vi "LSX Set Stop Accel.vi"(6 "dAD":dbl, 7 "dZD":dbl, 8 "error in (no error)":errorcluster, 9 "dYD":dbl, 10 "dXD":dbl, 11 "lLSID":i32) -> (0 "error out":errorcluster, 3 "function return":i32)   [LabVIEW 2018, in "Tango.lvlib"]
doc: "TANGOAPI int TANGOCALL LSX_SetStopAccel (int lLSID, double dXD, double dYD, double dZD, double dAD);"
uses:
  Tango.lvlib
  SubVIs/Tango_DLL.dll
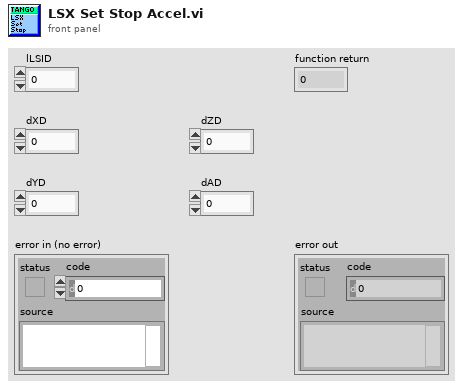
[diagram p1: front panel]
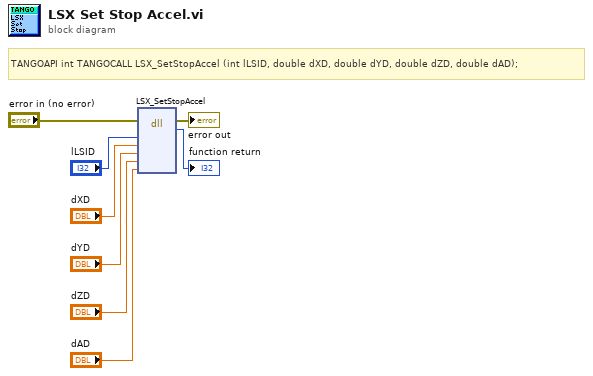
[diagram p0: block diagram]
diagram:
  # "TANGOAPI int TANGOCALL LSX_SetStopAccel (int lLSID, double dXD, double dYD, double dZD, double dAD);"
  n1 = dll-call lib="C:/Users/Familie/Documents/LabviewIX81/lib/TANGO Stage/SubVIs/Tango_DLL.*" fn="LSX_SetStopAccel"(error in="error in (no error)", "lLSID"="lLSID", "dXD"="dXD", "dYD"="dYD", "dZD"="dZD", "dAD"="dAD") -> (error out=→"error out":errorcluster, →"function return":i32)  [unwired: 7 in, 1 out]
